vi "MicroStrain 3DM-GXx Single Measurement.vi"() -> ()   [LabVIEW 2012]
doc: "Shows how to setup the device and acquire a single measurement."
uses:
  <instrlib>/MicroStrain 3DM-GXx/Public/Data/Read Single Measurement/Read (Euler Angles).vi
  <instrlib>/MicroStrain 3DM-GXx/MicroStrain 3DM-GXx.lvlib
panel:
  in  "VISA resource name":refnum<visa-resource-name>
  out "Yaw":dbl
  out "Pitch":dbl
  out "Roll":dbl
  out "Timer":dbl
  # "(c) 2009 - 2011 National Instruments.  ALL RIGHTS RESERVED."
  # "This VI demonstrates the process of requesting a single measurement from the device.\nThis example requests the Euler Angles measurement.  To request a different\nmeasurement simply change the selection on the 'Read Single Measurement' VI in \nthe block diagram and create indicators based on the new outputs of that VI."
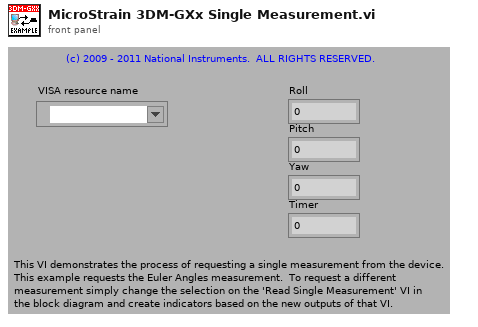
[diagram p1: front panel]
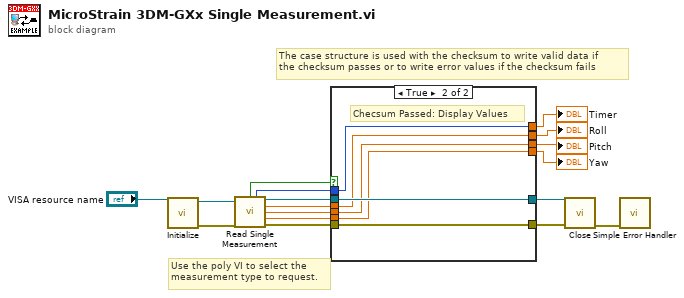
[diagram p0: block diagram]
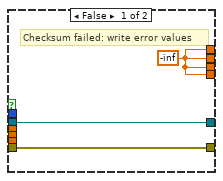
[diagram p2: hidden frame]
diagram:
  # "The case structure is used with the checksum to write valid data if \nthe checksum passes or to write error values if the checksum fails"
  # "Use the poly VI to select the \nmeasurement type to request."
  n1 = call <instrlib>:"Initialize.vi"("VISA resource name"="VISA resource name") -> ("error out"=w1:errorcluster, "VISA resource name out"=w2:refnum<visa-resource-name>)  [unwired: 9 in]
  n2 = call-poly <instrlib>:"Read Single Measurement.vi"("VISA resource name"=w2, "error in (no error)"=w1) -> ("Checksum Pass"=w9:bool, "Timer"=w8:u32, "VISA resource name out"=w16:refnum<visa-resource-name>, "Roll"=w15:sgl, "Pitch"=w14:sgl, "Yaw"=w13:sgl, "error out"=w12:errorcluster)  [unwired: 7 in]
  n3 = case shown="True" w9 {
    tunnel: w16 -> [w19 w26]
    tunnel: w15 -> [_ w24]
    tunnel: w14 -> [_ w23]
    tunnel: w13 -> [_ w22]
    tunnel: w12 -> [w18 w25]
    tunnel: [w19 w26] -> w11
    tunnel: [w18 w25] -> w10
    tunnel: [w20 w24] -> w6
    tunnel: [w20 w23] -> w5
    tunnel: [w20 w22] -> w4
    tunnel: w8 -> [_ w21]
    tunnel: [w20 w21] -> w7
    frame False {
      w20 = -inf
      # "Checksum failed: write error values"
    }
    frame True {
      # "Checsum Passed: Display Values"
    }
  }
  "Timer" <- w7
  "Roll" <- w6
  "Pitch" <- w5
  "Yaw" <- w4
  n4 = call <instrlib>:"Close.vi"("error in (no error)"=w10, "VISA resource name"=w11) -> ("error out"=w17:errorcluster)  [unwired: 9 in]
  n5 = call <vilib>:"Simple Error Handler.vi"("error in (no error)"=w17) -> ()  [unwired: 4 in, 5 out]
